vi "point thermal model 2.vi"(4 "Reset?":bool, 6 "dt":dbl=1.0 format="%0.2f", 8 "Ambient Temp":dbl=900.0, 9 "Sensor T0":dbl=25.0, 10 "Duty Cycle %":dbl=25.0, 11 "X":dbl[](array[numeric])) -> (2 "T":dbl)   [LabVIEW 2014, in "UEGO Sim Engine.lvlib"]
uses:
  UEGO Sim Engine.lvlib
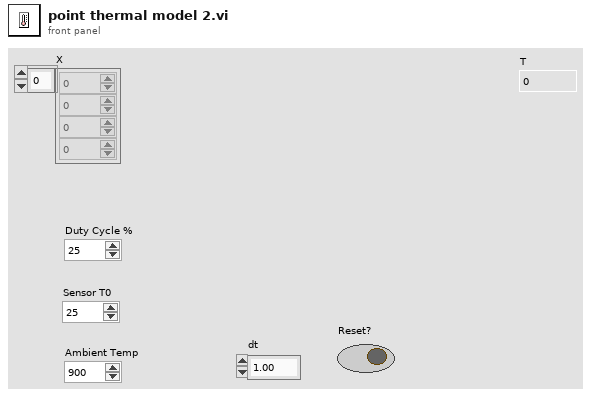
[diagram p1: front panel]
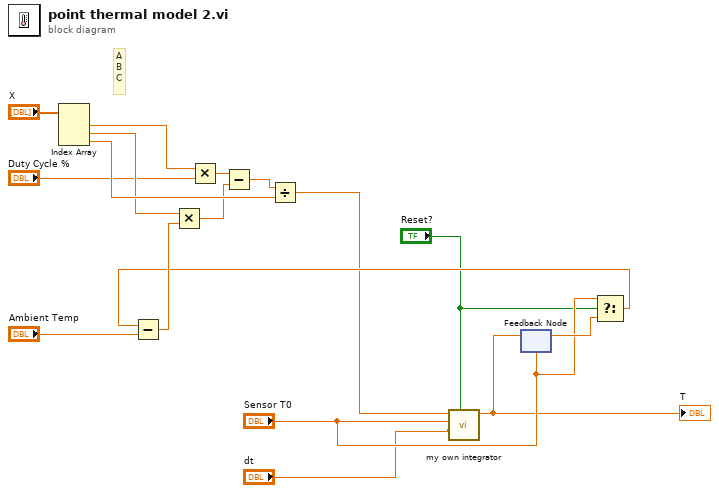
[diagram p0: block diagram]
diagram:
  # "A\nB\nC"
  n1 = Index Array(array="X") -> (element #1=w9:dbl, element #2=w13:dbl, element #3=w16:dbl)  [unwired: 3 in]
  n2 = Multiply ("Multiply 2")(x=w9, y="Duty Cycle %") -> (x*y=w11:dbl)
  n3 = feedback #1("Sensor T0") -> (w7:dbl)
  n4 = Select(t="Sensor T0", s="Reset?", f=w7) -> (s? t:f=w6:dbl)
  n5 = Subtract ("Subtract 2")(x=w6, y="Ambient Temp") -> (x-y=w14:dbl)
  n6 = Multiply(x=w13, y=w14) -> (x*y=w15:dbl)
  n7 = Subtract(x=w11, y=w15) -> (x-y=w17:dbl)
  n8 = Divide(x=w17, y=w16) -> (x/y=w5:dbl)
  n9 = call "my own integrator.vi"("initialize"="Reset?", "dt"="dt", "initial condition"="Sensor T0", "x"=w5) -> ("integral x(t)"=w1:dbl)  [unwired: 7 in]
  "T" <- w1
  n10 = feedback-in #1(w1) -> ()
